vi ".NET Type Builder Define Field.vi"(8 "error in (no error)":errorcluster, 9 ".NET Type Builder":refnum<k24>, 10 ".NET Type":refnum<k24>, 11 "Name":string) -> (0 "error out":errorcluster, 1 ".NET Field Builder":refnum<k24>)   [LabVIEW 2018, in "TwinCAT ADS.lvclass"]
uses:
  TwinCAT ADS.lvclass
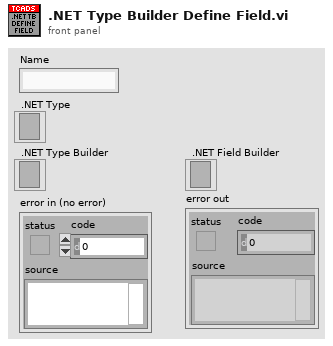
[diagram p1: front panel]
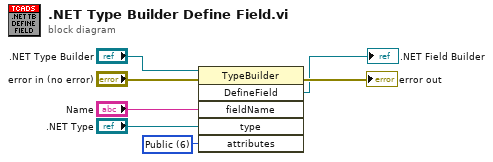
[diagram p0: block diagram]
diagram:
  w3 = 6 items=["PrivateScope"=0, "Private"=1, "FamANDAssem"=2, "Assembly"=3, "Family"=4, "FamORAssem"=5, "Public"=6, "FieldAccessMask"=7, "Static"=16, "InitOnly"=32, "Literal"=64, "NotSerialized"=128, "HasFieldRVA"=256, "SpecialName"=512, "RTSpecialName"=1024, "HasFieldMarshal"=4096, "PinvokeImpl"=8192, "HasDefault"=32768, "ReservedMask"=38144] ("attributes")
  n1 = invoke class="TypeBuilder" method="DefineField"(reference=".NET Type Builder", error in="error in (no error)", "fieldName"="Name", "type"=".NET Type", "attributes"=w3) -> (error out=→"error out":errorcluster, "DefineField"=→".NET Field Builder":refnum<k24>)  [unwired: 1 in, 4 out]
